vi "Detector Test.vi"() -> ()   [LabVIEW 2020]
uses:
  <vilib>/Utility/error.llb/DialogType.ctl
  TALOS/TALOS_PPL.lvlibp/Classes/Father of all Detectors/Father Of All Detectors.lvclass
  TALOS/TALOS_PPL.lvlibp/Internal uServices/System uServices/Detector Manager/Detector Manager/Detector Manager.lvclass
panel:
  in  "Stop":bool
  in  "Timeout (s)":dbl
  in  "Parameter Selector":string
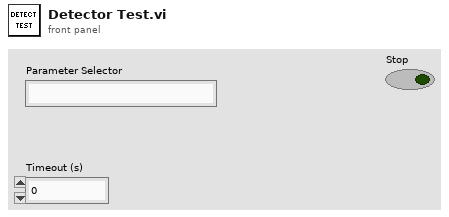
[diagram p1: front panel]
types:
  T1 = typedef "DialogType.ctl" = u16
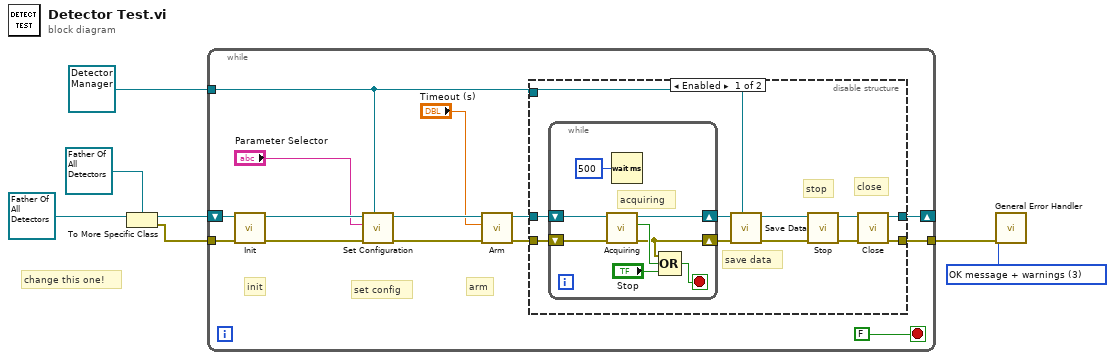
[diagram p0: block diagram]
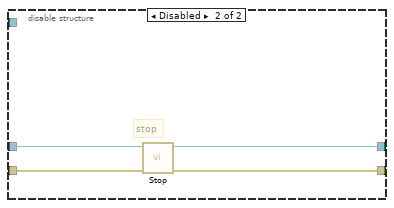
[diagram p2: hidden frame]
diagram:
  w6 = T1 3 items=["no dialog", "OK message", "continue or stop message", "OK message + warnings", "continue/stop + warnings"] ("type of dialog (OK msg:1)")
  # "change this one!"
  n1 = To More Specific Class(target class=refnum<class "Father Of All Detectors.lvclass"> refnum ("TALOS_PPL.lvlibp:Father Of All Detectors.lvlib:Father Of All Detectors.lvclass"), reference=refnum<class "Father Of All Detectors.lvclass"> refnum ("TALOS_PPL.lvlibp:Father Of All Detectors.lvlib:Father Of All Detectors.lvclass")) -> (specific class reference=w4:refnum<class "Father Of All Detectors.lvclass">, error out=w5:errorcluster)  [unwired: 1 in]
  n2 = while {
    shift-right: [w19] -> _
    shift-left: w4 -> [w18]
    tunnel: w5 -> [w17]
    tunnel: [w21] -> w7
    tunnel: refnum<class "Detector Manager.lvclass"> refnum ("TALOS_PPL.lvlibp:Detector Manager.lvlib:Detector Manager.lvclass") -> [w8]
    stop <- FALSE stop-if-true
    # "arm"
    # "set config"
    # "init"
    n3 = call-dynamic "Init.vi"("error in (no error)"=w17, "Father Of All Detectors in"=w18) -> ("error out"=w15:errorcluster, "Father Of All Detectors out"=w16:refnum<class "Father Of All Detectors.lvclass">)  [unwired: 7 in, 1 out]
    n4 = call-dynamic "Set Configuration.vi"("Detector Manager"=w8, "error in (no error)"=w15, "Configuration Name"="Parameter Selector", "Father Of All Detectors in"=w16) -> ("error out"=w12:errorcluster, "Father Of All Detectors out"=w13:refnum<class "Father Of All Detectors.lvclass">)  [unwired: 6 in]
    n5 = call-dynamic "Arm.vi"("error in (no error)"=w12, "Timeout (s)"="Timeout (s)", "Father Of All Detectors in"=w13) -> ("error out"=w9:errorcluster, "Father Of All Detectors out"=w10:refnum<class "Father Of All Detectors.lvclass">)  [unwired: 6 in, 1 out]
    n6 = disable-structure shown="Enabled" {
      disable-tunnel: w10 -> [w32 w41]
      disable-tunnel: w9 -> [w31 w44]
      disable-tunnel: [w25 w43] -> w21
      disable-tunnel: [w22 w42] -> w19
      disable-tunnel: w8 -> [w29 _]
      frame Enabled {
        # "close"
        # "stop"
        # "save data"
        n7 = while {
          shift-right: [w35] -> w30
          shift-left: w32 -> [w36]
          shift-right: [w33] -> w28
          shift-left: w31 -> [w37]
          stop <- w40 stop-if-true
          # "acquiring"
          n8 = call-dynamic "Acquiring.vi"("error in (no error)"=w37, "Father Of All Detectors in"=w36) -> ("error out"=w33:errorcluster, "Ready to Save Data?"=w34:bool, "Father Of All Detectors out"=w35:refnum<class "Father Of All Detectors.lvclass">)  [unwired: 7 in]
          n9 = Wait (ms)(milliseconds to wait=u32 500) -> ()  [unwired: 1 out]
          n10 = Compound Arithmetic op=OR(w33, w34, "Stop") -> (w40:bool)
        }
        n11 = call-dynamic "Save Data.vi"("Detector Manager"=w29, "error in (no error)"=w28, "Father Of All Detectors in"=w30) -> ("error out"=w27:errorcluster, "Father Of All Detectors out"=w24:refnum<class "Father Of All Detectors.lvclass">)  [unwired: 6 in, 1 out]
        n12 = call-dynamic "Stop.vi"("error in (no error)"=w27, "Father Of All Detectors in"=w24) -> ("error out"=w26:errorcluster, "Father Of All Detectors out"=w23:refnum<class "Father Of All Detectors.lvclass">)  [unwired: 8 in]
        n13 = call-dynamic "Close.vi"("error in (no error)"=w26, "Father Of All Detectors in"=w23) -> ("error out"=w25:errorcluster, "Father Of All Detectors out"=w22:refnum<class "Father Of All Detectors.lvclass">)  [unwired: 8 in]
      }
      frame Disabled {
        # "stop"
        n14 = call-dynamic "Stop.vi"("error in (no error)"=w44, "Father Of All Detectors in"=w41) -> ("error out"=w43:errorcluster, "Father Of All Detectors out"=w42:refnum<class "Father Of All Detectors.lvclass">)  [unwired: 8 in]
      }
    }
  }
  n15 = call <vilib>:"General Error Handler.vi"("type of dialog (OK msg:1)"=w6, "error in (no error)"=w7) -> ()  [unwired: 9 in, 5 out]
